vi "Variable list Modem Status digital.vi"() -> (6 "Variant":variant, 10 "Array":T1[](array[typedef]))   [LabVIEW 2011]
uses:
  Measurments Handling/Fixed Digital Channel Definition.ctl
  Measurments Handling/Update frequensies.ctl
  Measurments Handling/Channel catagory Enum.ctl
  Variable List Modem Status Digital.ctl
  Measurments Handling/Common/Variable List Common Digital.ctl
  Tool/Variable List Tool Digital.ctl
  <vilib>/Utility/VariantDataType/GetNumericInfo.vi
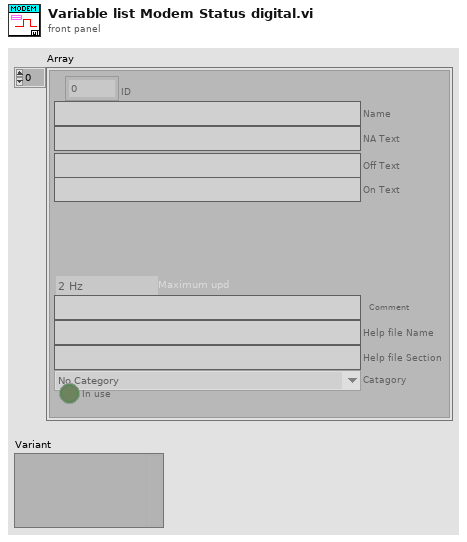
[diagram p1: front panel]
types:
  T1 = typedef "Fixed Digital Channel Definition.ctl" = cluster{"ID":u16, "Name":string, "NA Text":string, "Off Text":string, "On Text":string, "Maximum upd":T2, "Comment":string, "Help file Name":string, "Help file Section ":string, "Catagory":T3, "In use":bool}
  T2 = typedef "Update frequensies.ctl" = enum16{"2 Hz", "1 Hz", "0.1 Hz"}
  T3 = typedef "Channel catagory Enum.ctl" = enum16{"No Category", "Power", "Temperature", "Pressure"}
  T4 = typedef "Variable List Tool Digital.ctl" = enum16{"Tool Error Controller", "Tool Stopped Controller", "Tool Relay 1", "Tool Relay 2", "Tool Both Relays", "Tool node Pressure 1", "Tool Error Pressure 1", "Tool Stopped Pressure 1", "Tool node Pressure 2", "Tool Error Pressure 2", "Tool Stopped Pressure 2", "Tool node Solenoid", "Tool Error Solenoid", "Tool Stopped Solenoid", "Tool Solenoid 1", "Tool Solenoid 2", "Tool Solenoid 3", "Tool node PSU", "Tool Error PSU", "Tool Stopped PSU", "Upper Tension Sub", "Tool Error Upper Tension Sub", "Tool Stopped Upper Tension Sub", "Lower Tension Sub", "Tool Error Lower Tension Sub", "Tool Stopped Lower Tension Sub", "Stroke Target seeking", "Stroke Moving Out", "Stroke Moving Inn", "Stroke valves set for Out", "Stroke valves set for In", "Stroke In (force)", "Stroke Out (force)", "Stroke Force decreasing(in)", "Stroke Force decreasing(out)", "Stroke Force change not correct", "Stroke SLIPS established P1", "Stroke SLIPS established P2", "Stroke SLIPS established", "Stroke Pressure Monitor Ongoing", "Stroke Pressure Monitor Ending ", "Tool Stroke enable Valve", "Tool Stroke direction Valve", "Tool Anchor Valve", "Stroker Var19 - Reserved", "Stroker Var20 - Reserved", "Stroker Var21 - Reserved", "Stroker Var22 - Reserved", "Stroker Var23 - Reserved", "Stroker Var24 - Reserved", "Tractor Var1 - Reserved", "Tractor Var2 - Reserved", "Tractor Var3 - Reserved", "Tractor Var4 - Reserved", "Tractor Var5 - Reserved", "Tractor Var6 - Reserved", "Tractor Var7 - Reserved", "Tractor Var8 - Reserved", "Oil filling mode", "Mill Bit Direction", "Position control", "Anchor", "Driller Var5 - Reserved", "Driller Var6 - Reserved", "Driller Var7 - Reserved", "Driller Var8 - Reserved"}
  T5 = typedef "Variable List Common Digital.ctl" = enum16{"PCP Connected", "PCP PC Control", "HV PSU connected", "HV PSU HV Active", "Modem Connected", "Tool Connected", "CanBus interface"}
  T6 = typedef "Variable List Modem Status Digital.ctl" = enum16{"TMU_LINK_STATUS"}
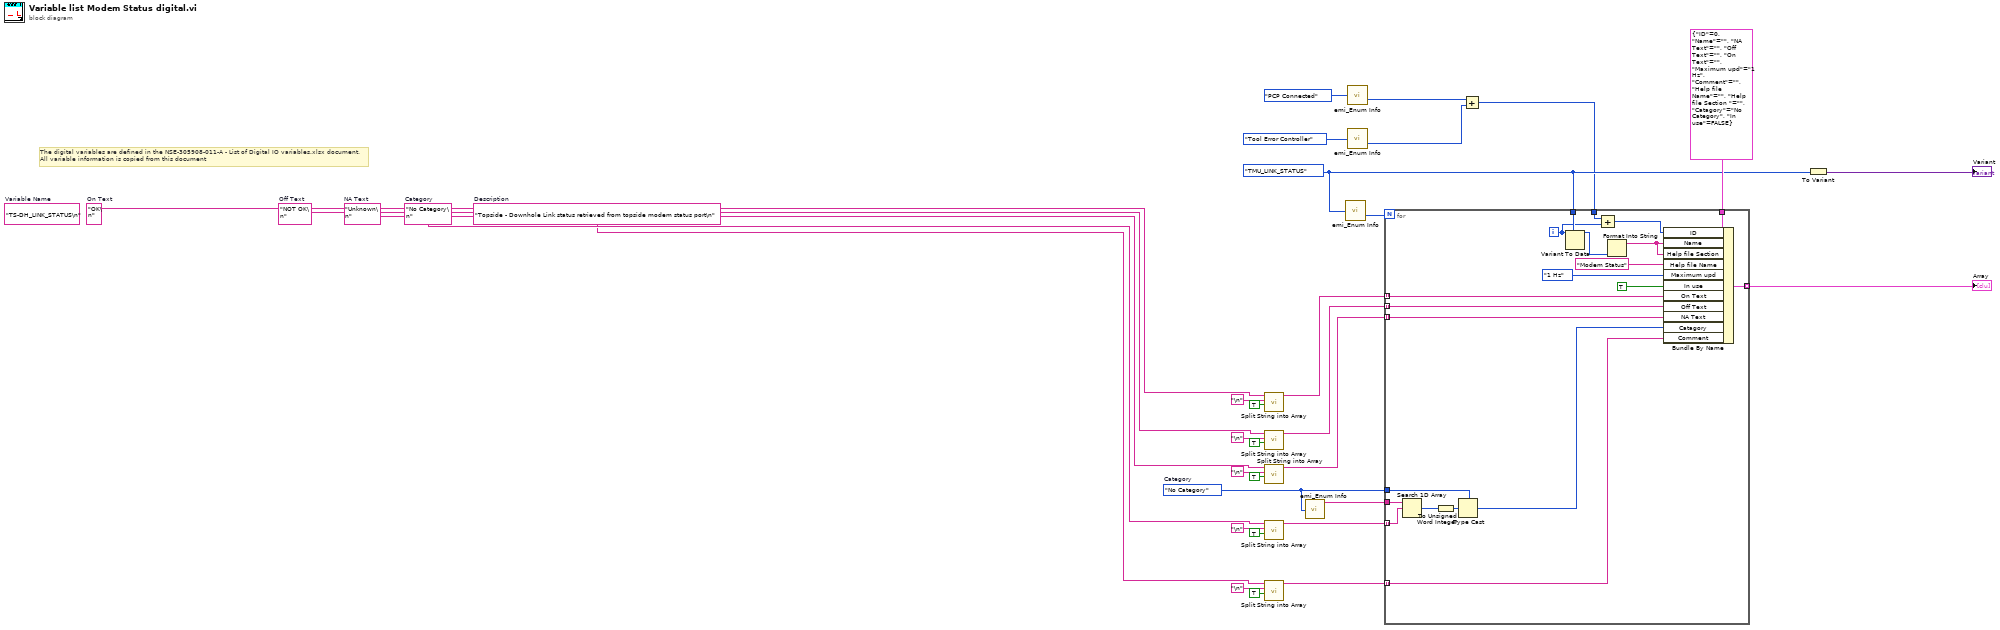
[diagram p0: block diagram]
diagram:
  w6 = Variable_List_Modem_Status_Digital."TMU_LINK_STATUS"
  w9 = Channel_catagory_Enum."No Category"  # Category
  w15 = "No Category\n"  # Category
  w7 = "Topside - Downhole Link status retrieved from topside modem status port\n"  # Description
  w20 = "Unknown\n"  # NA Text
  w23 = "NOT OK\n"  # Off Text
  w26 = "OK\n"  # On Text
  (unwired) "TS-DH_LINK_STATUS\n"  # Variable Name
  # "The digital variables are defined in the NSE-305908-011-A - List of Digital IO variables.xlsx document.\nAll variable information is copied from this document"
  n1 = call "Split String into Array.vi"("Remove Last Row"=TRUE, "Separator"="\n", "Input string"=w26) -> ("Array of cells"=w14:string[])  [unwired: 8 in]
  n2 = call "Split String into Array.vi"("Remove Last Row"=TRUE, "Separator"="\n", "Input string"=w23) -> ("Array of cells"=w13:string[])  [unwired: 8 in]
  n3 = call "Split String into Array.vi"("Remove Last Row"=TRUE, "Separator"="\n", "Input string"=w20) -> ("Array of cells"=w12:string[])  [unwired: 8 in]
  n4 = call "Split String into Array.vi"("Remove Last Row"=TRUE, "Separator"="\n", "Input string"=w15) -> ("Array of cells"=w11:string[])  [unwired: 8 in]
  n5 = call "Split String into Array.vi"("Remove Last Row"=TRUE, "Separator"="\n", "Input string"=w7) -> ("Array of cells"=w8:string[])  [unwired: 8 in]
  n6 = call "emi_Enum Info.vi"("Enum"=w9) -> ("Text Elements"=w10:string[])  [unwired: 11 in, 3 out]
  n7 = call "emi_Enum Info.vi"("Enum"=w6) -> ("Numb Elements"=w30:i32)  [unwired: 11 in, 3 out]
  n8 = call "emi_Enum Info.vi"("Enum"=Variable_List_Common_Digital."PCP Connected" ("Action")) -> ("Numb Elements"=w3:i32)  [unwired: 11 in, 3 out]
  n9 = call "emi_Enum Info.vi"("Enum"=Variable_List_Tool_Digital."Tool Error Controller") -> ("Numb Elements"=w2:i32)  [unwired: 11 in, 3 out]
  n10 = Add(x=w3, y=w2) -> (x+y=w1:i32)
  n11 = for {
    N: w30 -> [_]
    tunnel: w6 -> [w35]
    tunnel: T1 {"ID"=0, "Name"="", "NA Text"="", "Off Text"="", "On Text"="", "Maximum upd"=enum."1 Hz", "Comment"="", "Help file Name"="", "Help file Section "="", "Catagory"=enum."No Category", "In use"=FALSE} ("Variable Defenition") -> [w51]
    tunnel: [w52] -> w31 mode=indexing
    tunnel: w14 -> [w46] mode=indexing
    tunnel: w13 -> [w45] mode=indexing
    tunnel: w12 -> [w44] mode=indexing
    tunnel: w11 -> [w41] mode=indexing
    tunnel: w10 -> [w40]
    tunnel: w9 -> [w39]
    tunnel: w8 -> [w37] mode=indexing
    tunnel: w1 -> [w36]
    i -> [w34]
    n12 = Search 1D Array(1D array=w40, element=w41) -> (index of element=w43:i32)  [unwired: 1 in]
    n13 = To Unsigned Word Integer(number=w43) -> (unsigned 16bit integer=w42:u16)
    n14 = Type Cast(type=w39, x=w42) -> (*(type *) &x=w38:T3)
    n15 = Variant To Data(type=w35, Variant=w34) -> (data=w53:T6)  [unwired: 1 in, 1 out]
    n16 = Add(x=w36, y=w34) -> (x+y=w33:i32)
    n17 = Format Into String(w53) -> (resulting string=w50:string)  [unwired: 3 in, 1 out]
    n18 = Bundle By Name(cluster=w51, "ID"=w33, "Name"=w50, "Help file Section"=w50, "Help file Name"="Modem Status", "Maximum upd"=Update_frequensies."1 Hz", "In use"=TRUE, "On Text"=w46, "Off Text"=w45, "NA Text"=w44, "Catagory"=w38, "Comment"=w37) -> (w52:T1)
  }
  "Array" <- w31
  n19 = To Variant(anything=w6) -> (Variant=→"Variant":variant)
